vi "Pre Launch Init.vi"(11 "TCPIP Communications in":refnum<class "TCPIP Communications.lvclass">) -> (0 "error out":errorcluster, 3 "TCPIP Communications out":refnum<class "TCPIP Communications.lvclass">)   [LabVIEW 2015, in "TCPIP Communications Framework.lvlib" / "TCPIP Communications.lvclass"]
doc: "(<B>Filename</B>: Actor Framework.lvlib:Actor.lvclass:Pre Launch Init.vi)\n\nDefines behavior that occurs after the Launch Nested Actor method is invoked but before the actor's Actor Core method begins running.\n\nBy default, this method does nothing. A descendant class may override it to define behavior."
uses:
  TCPIP Communications.lvclass
  TCPIP Communications.lvclass/TCPIP Communications.ctl
  <vilib>/ActorFramework/Actor/Actor.lvclass
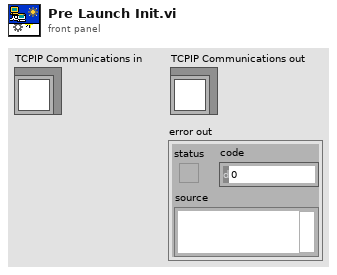
[diagram p1: front panel]
types:
  T1 = typedef "TCPIP Communications Framework.lvlib/TCPIP Communications.lvclass/notifiers cluster.ctl" = cluster{"stop":refnum<notifier>}
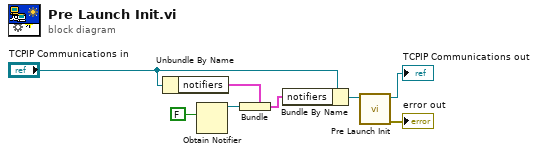
[diagram p0: block diagram]
diagram:
  n1 = Unbundle By Name("TCPIP Communications in") -> ("notifiers"=w4:T1)
  n2 = Obtain Notifier(notification data type=FALSE) -> (notifier out=w2:refnum<notifier>)  [unwired: 3 in, 2 out]
  n3 = Bundle(cluster=w4, "stop"=w2) -> (w3:T1)
  n4 = Bundle By Name(cluster="TCPIP Communications in", "notifiers"=w3) -> (w5:refnum<class "TCPIP Communications.lvclass">)
  n5 = call-parent "Pre Launch Init.vi"("Actor in"=w5) -> ("error out"=→"error out":errorcluster, "Actor out"=→"TCPIP Communications out":refnum<class "TCPIP Communications.lvclass">)  [unwired: 9 in]
